vi "Destroy.vi"(0 "reference in":refnum<class "MyClass1_IMyInterface.lvclass">, 5 "error in (no error)":errorcluster) -> (14 "reference out":refnum<class "MyClass1_IMyInterface.lvclass">, 19 "error out":errorcluster)   [LabVIEW 2017, in "MyClass1_IMyInterface.lvclass"]
doc: "Destructor."
uses:
  MyClass1_IMyInterface.lvclass
  IMyInterface_interface/IMyInterface.lvclass
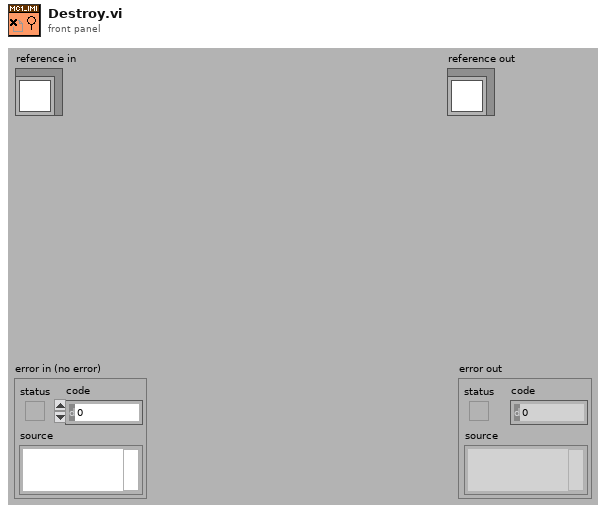
[diagram p1: front panel]
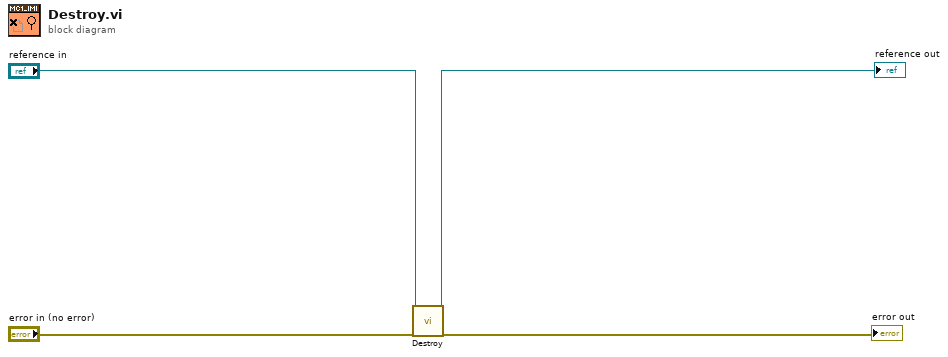
[diagram p0: block diagram]
diagram:
  n1 = call-parent "Destroy.vi"("reference in"="reference in", "error in (no error)"="error in (no error)") -> ("reference out"=→"reference out":refnum<class "MyClass1_IMyInterface.lvclass">, "error out"=→"error out":errorcluster)  [unwired: 16 in]
